vi "Reciver.vi"(8 "Error In":errorcluster, 11 "Ref boolean in":refnum<vi>) -> (0 "Error Out":errorcluster)   [LabVIEW 2020]
uses:
  Ctrls/GlobalStop.vi
panel:
  out "Data Chart":dbl(graph)
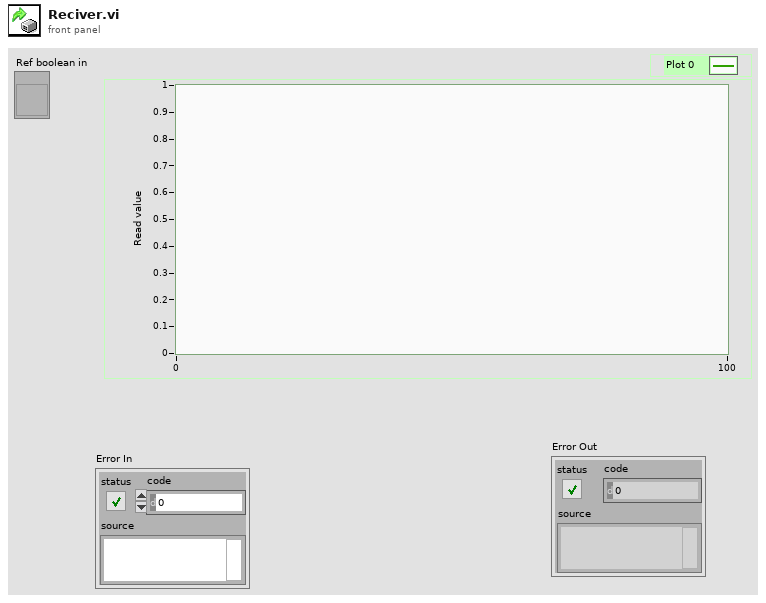
[diagram p1: front panel]
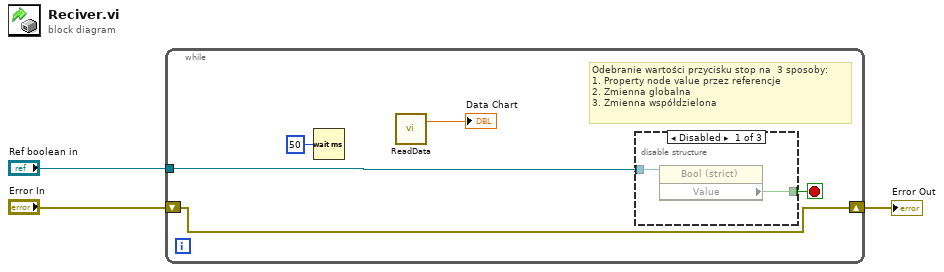
[diagram p0: block diagram]
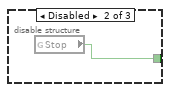
[diagram p2: hidden frame]
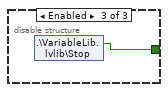
[diagram p3: hidden frame]
diagram:
  n1 = while {
    tunnel: "Ref boolean in" -> [w5]
    shift-right: [w4] -> w1
    shift-left: "Error In" -> [w4]
    stop <- w8 stop-if-true
    # "Odebranie wartości przycisku stop na  3 sposoby:\n1. Property node value przez referencje\n2. Zmienna globalna\n3. Zmienna współdzielona"
    n2 = Wait (ms)(milliseconds to wait=u32 50) -> ()  [unwired: 1 out]
    n3 = call "ReadData.vi"() -> ("number: 0 to 1"=→"Data Chart":dbl)  [unwired: 3 in]
    n4 = disable-structure shown="Disabled" {
      disable-tunnel: [w9 w11 w12] -> w8
      disable-tunnel: w5 -> [w10 _ _]
      frame Disabled {
        n5 = property on="Property Node" class="Bool (strict)"(reference=w10) -> ("Value"=w9:bool)  [unwired: 1 in, 2 out]
      }
      frame Disabled {
        n6 = global read "GlobalStop.vi" "Stop"() -> (w11:bool)
      }
      frame Enabled {
        n7 = shared-variable ".\\VariableLib.lvlib\\Stop"() -> (w12:bool)  [unwired: 1 in, 1 out]
      }
    }
  }
  "Error Out" <- w1
